vi "main.vi"() -> ()   [LabVIEW 2014]
doc: "Use this template to build a producer/consumer design pattern with events to produce queue items. Use this design pattern instead of the User Interface Event Handler pattern for user interfaces when you want to execute code asynchronously in response to an event without slowing the user interface responsiveness."
uses:
  Standard VISA Connection Template/VISA Connection Template.lvlib
panel:
  in  "Init_api":bool
  out "Device connected":refnum<visa-resource-name>
  in  "stop":bool
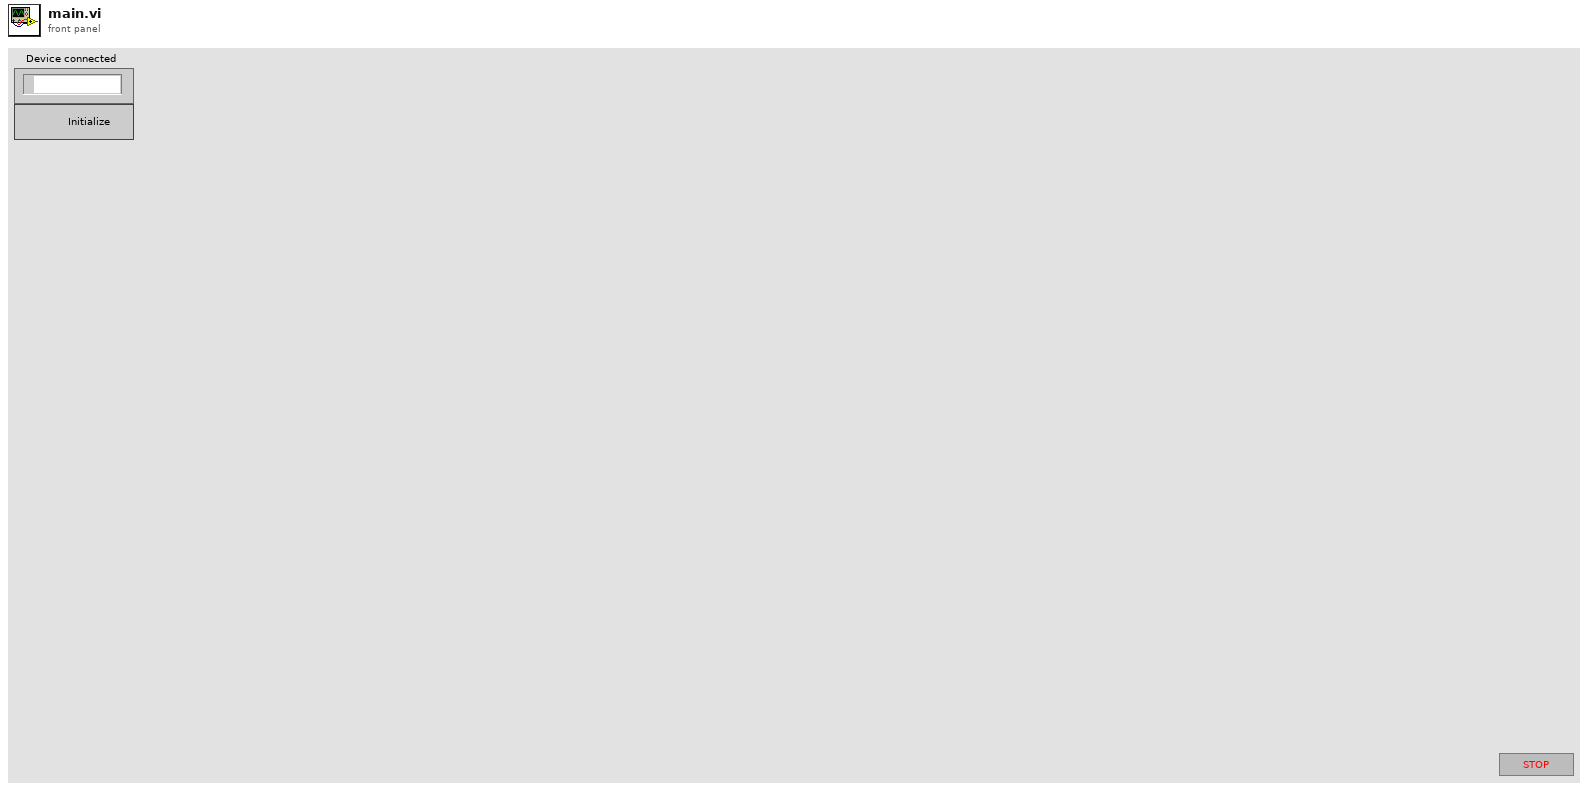
[diagram p1: front panel]
types:
  T1 = cluster{"port":refnum<visa-resource-name>, "Buff":string}
  T2 = typedef "Control 1" = enum16{"Initialize"}
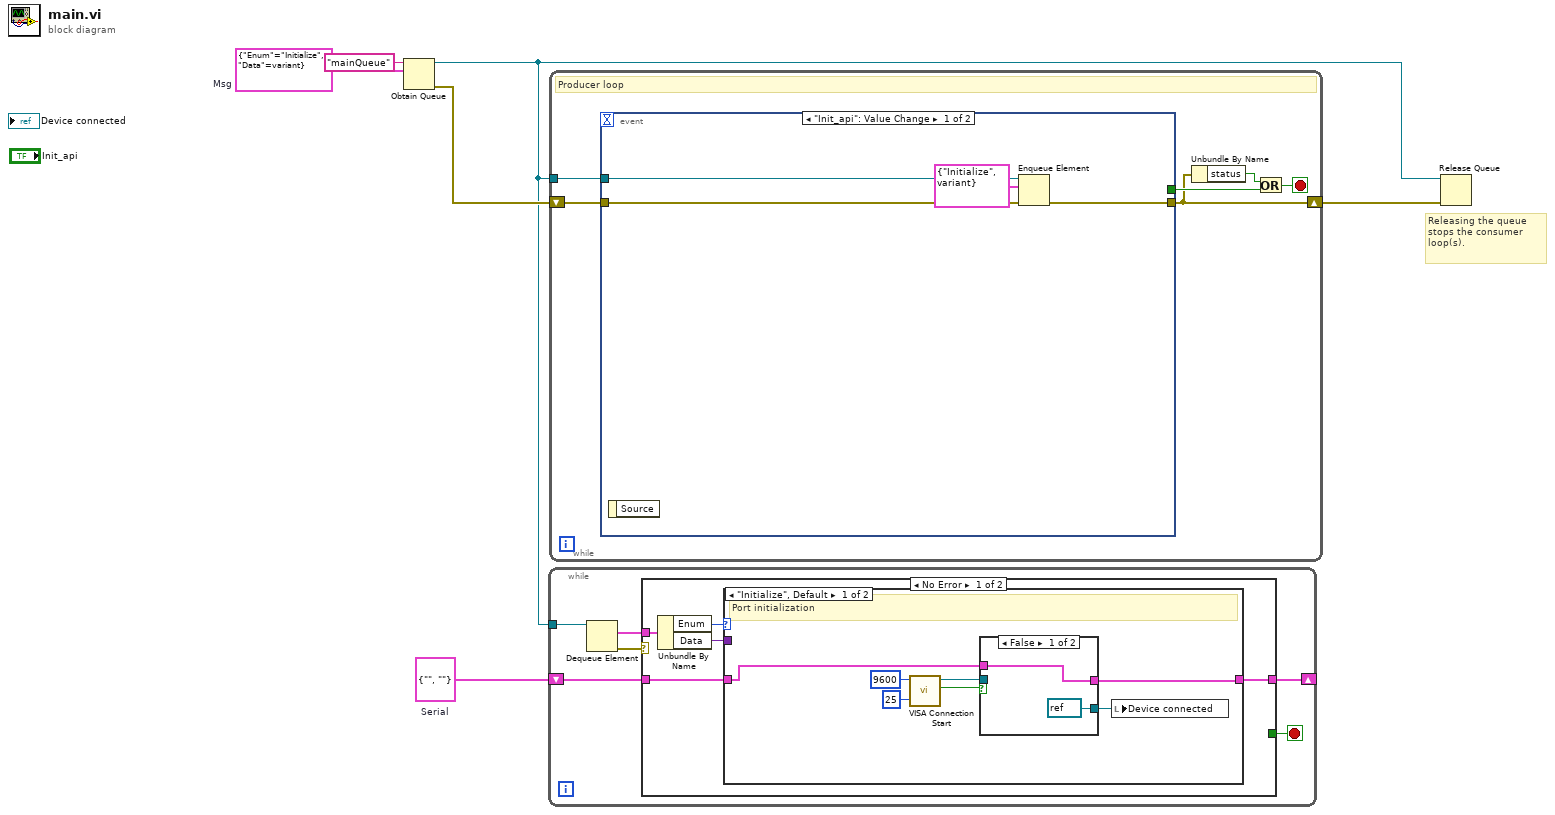
[diagram p0: block diagram]
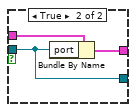
[diagram p2: hidden frame]
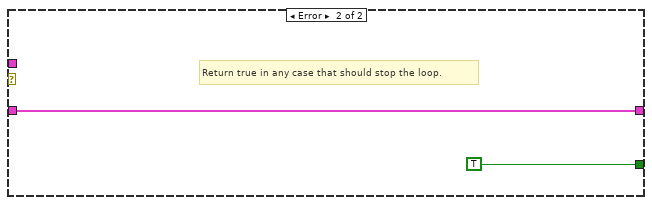
[diagram p4: hidden frame]
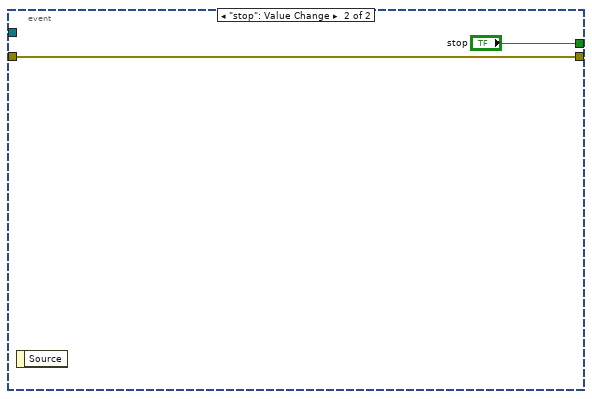
[diagram p5: hidden frame]
diagram:
  w1 = T1 {"port"="", "Buff"=""}  # Serial
  w3 = cluster{"Enum":T2, "Data":variant} {"Enum"=enum."Initialize", "Data"=variant}  # Msg
  # "Releasing the queue stops the consumer loop(s)."
  n1 = Obtain Queue(name (unnamed)="mainQueue", element data type=w3) -> (queue out=w4:refnum<queue>, error out=w6:errorcluster)  [unwired: 3 in, 1 out]
  n2 = while {
    tunnel: w4 -> [w12]
    shift-right: [w7] -> _
    shift-left: w1 -> [w8]
    stop <- w9 stop-if-true
    n3 = Dequeue Element(queue=w12) -> (element=w10:cluster{"Enum":T2, "Data":variant}, error out=w11:errorcluster)  [unwired: 2 in, 2 out]
    n4 = case shown="No Error" w11 {
      tunnel: w10 -> [w17 _]
      tunnel: [_ TRUE] -> w9
      tunnel: w8 -> [w14 w31]
      tunnel: [w13 w31] -> w7
      frame No Error {
        n5 = Unbundle By Name(w17) -> ("Enum"=w16:T2, "Data"=w15:variant)
        n6 = case shown="\"Initialize\", Default" w16 {
          tunnel: w15 -> [_ _]
          tunnel: w14 -> [w22 w30]
          tunnel: [w20 w30] -> w13
          frame "Initialize", Default {
            # "Port initialization"
            n7 = call "VISA Connection Start.vi"("Ports to search"=25, "Baud"=9600) -> ("Found?"=w19:bool, "VISA resource name"=w21:refnum<visa-resource-name>)  [unwired: 5 in, 1 out]
            n8 = case shown="False" w19 {
              tunnel: w22 -> [w26 w29]
              tunnel: w21 -> [_ w27]
              tunnel: [w26 w28] -> w20
              tunnel: [refnum<visa-resource-name> refnum ("VISA resource name") w27] -> w18
              frame False {
              }
              frame True {
                n9 = Bundle By Name(cluster=w29, "port"=w27) -> (w28:T1)
              }
            }
            n10 = local write "Device connected"(w18) -> ()
          }
          frame "Initialize" {
            # "State Machine"
          }
        }
      }
      frame Error {
        # "Return true in any case that should stop the loop."
      }
    }
  }
  n11 = while {
    shift-right: [w34] -> w5
    shift-left: w6 -> [w37]
    tunnel: w4 -> [w38]
    stop <- w35 stop-if-true
    # "Producer loop"
    n12 = event shown="[0] \"Init_api\": Value Change" {
      selector: _ -> [_ _]
      dyn-events: _ -> [_ _]
      timeout: _ -> [_ _]
      tunnel: w38 -> [w42 _]
      tunnel: w37 -> [w41 w43]
      tunnel: [w40 w43] -> w34
      tunnel: [_ "stop"] -> w36
      event "Init_api": Value Change {
        n13 = event-data() -> ()  [unwired: 1 in, 1 out]
        n14 = Enqueue Element(queue=w42, element=cluster{"Enum":T2, "Data":variant} {"Enum"=enum."Initialize", "Data"=variant}, error in (no error)=w41) -> (error out=w40:errorcluster)  [unwired: 1 in, 2 out]
      }
      event "stop": Value Change {
        n15 = event-data() -> ()  [unwired: 1 in, 1 out]
      }
    }
    n16 = Unbundle By Name(w34) -> ("status"=w33:bool)
    n17 = Or(x=w33, y=w36) -> (x .or. y?=w35:bool)
  }
  n18 = Release Queue(queue=w4, error in (no error)=w5) -> ()  [unwired: 1 in, 3 out]
